vi "Graphe 3D_Qua2ray.vi"(4 "Nbre colonnes":i8=4 min=1, 5 "file path (dialog if empty)":path caption="chemin du fichier (boîte de dialogue si vide)", 7 "Nbre lignes entête":i8=2 min=1, 8 "N° colonne Y":i8=2 min=1, 9 "N° colonne X":i8=1 min=1) -> ()   [LabVIEW 2013]
uses:
  <vilib>/Platform/NI_3dgraph.lvlib
  <vilib>/Analysis/NI_AALBase.lvlib
panel:
  out "Go":bool
  in  "Init Vue":bool
  in  "Plan - Vue":i32(ring)=3 items=["Plan XY", "Plan XZ", "Plan YZ", "Vue 3D"]
  in  "System Link Text 4":bool
  in  "System Link Text 3":bool
  out "Ecart type":dbl caption="Ecart-type" format="%0.2f"
  in  "System Link Text 2":bool
  in  "System Link Text":bool
  out "Min":dbl
  out "Max":dbl
  out "Moyenne":dbl format="%0.2f"
  in  "Inverser échelle Y":bool caption="Y"
  in  "Inverser échelle x":bool caption="X"
  in  "Plot Style":i32(ring)=5 caption="Style de courbe" items=["Ligne"=1, "Point"=2, "Ligne - Point"=3, "Maillage"=4, "Surface"=5, "Surface - Ligne"=6, "Surface Normale"=7, "Contour Ligne"=8, "Surface Contour"=9]
  in  "Transparency (%)":dbl(slide) caption="Transparence (%)" scale=0.0..80.0
  in  "Quit":bool
  in  "Paramètre":u16(ring)
  in  "3D Surface 4":refnum<k7>(container) caption="Surface en 3D"
  in  "3D Surface 3":refnum<k7>(container) caption="Surface en 3D"
  in  "3D Surface 2":refnum<k7>(container) caption="Surface en 3D"
  in  "3D Surface":refnum<k7>(container) caption="Surface en 3D"
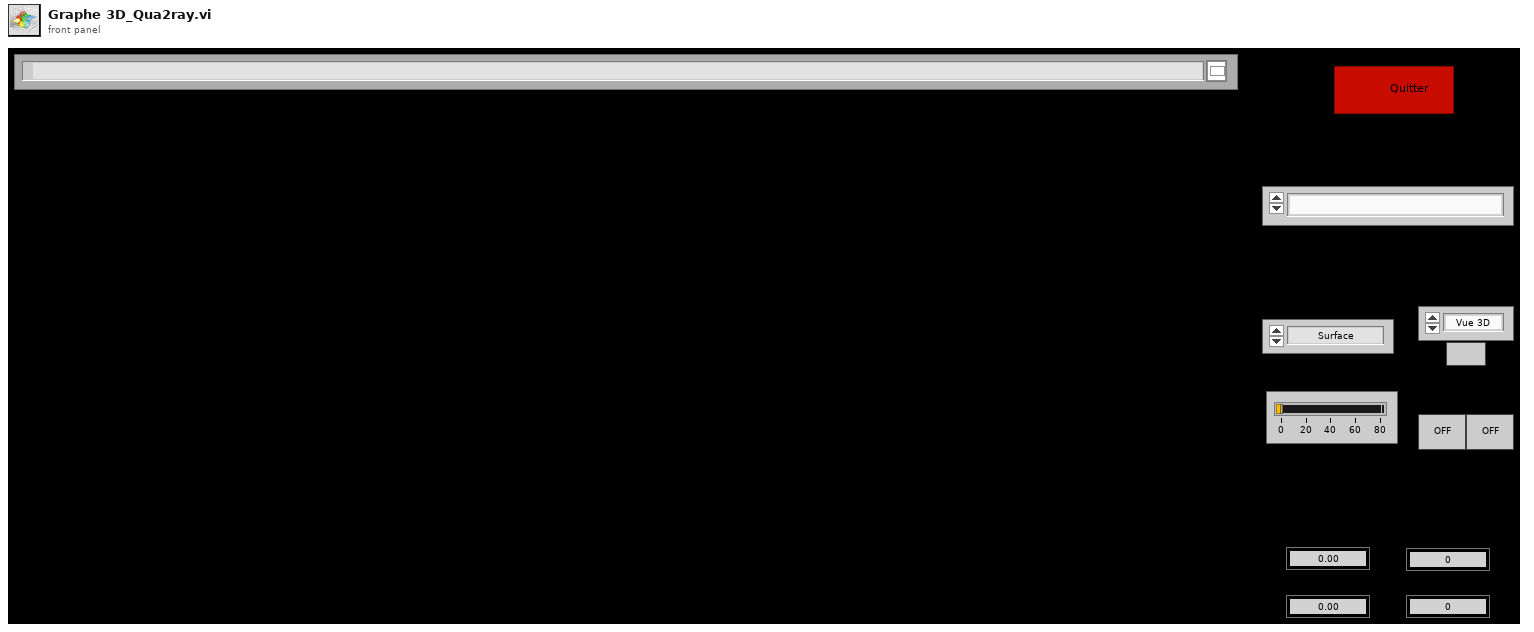
[diagram p1: front panel]
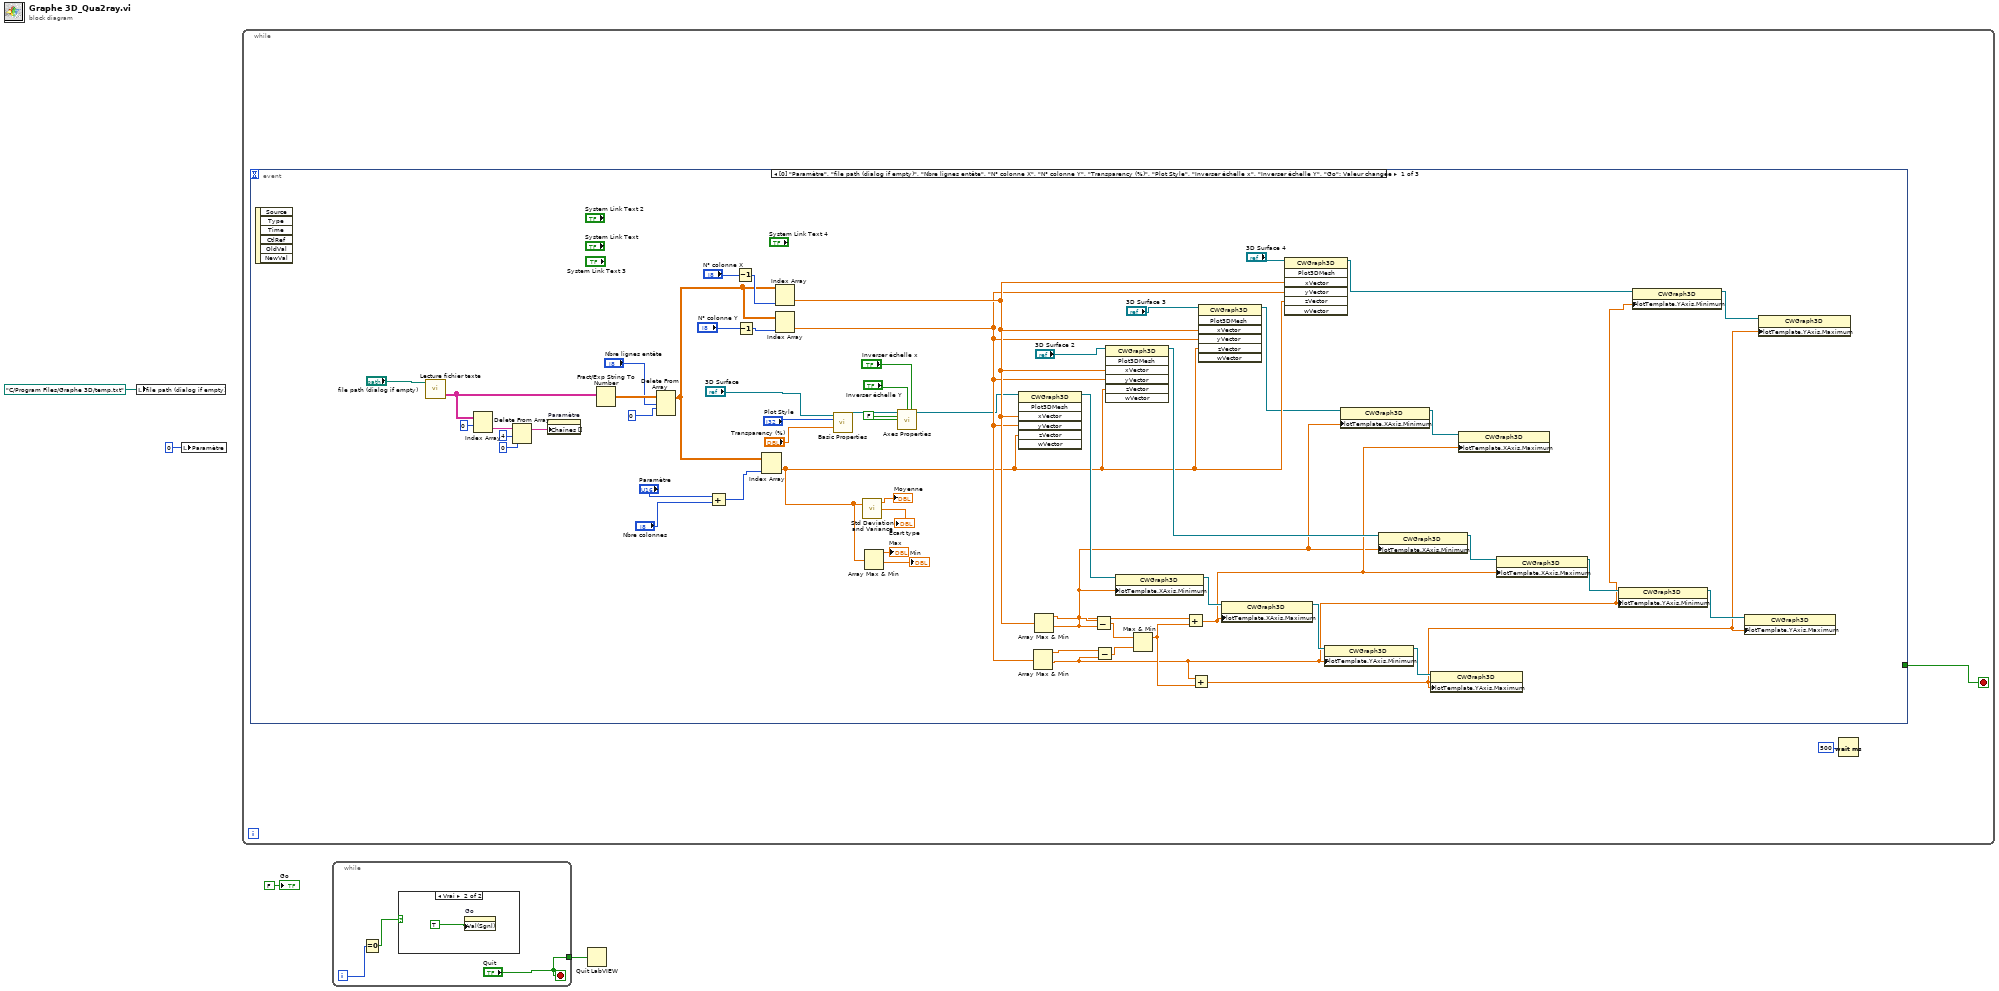
[diagram p0: block diagram]
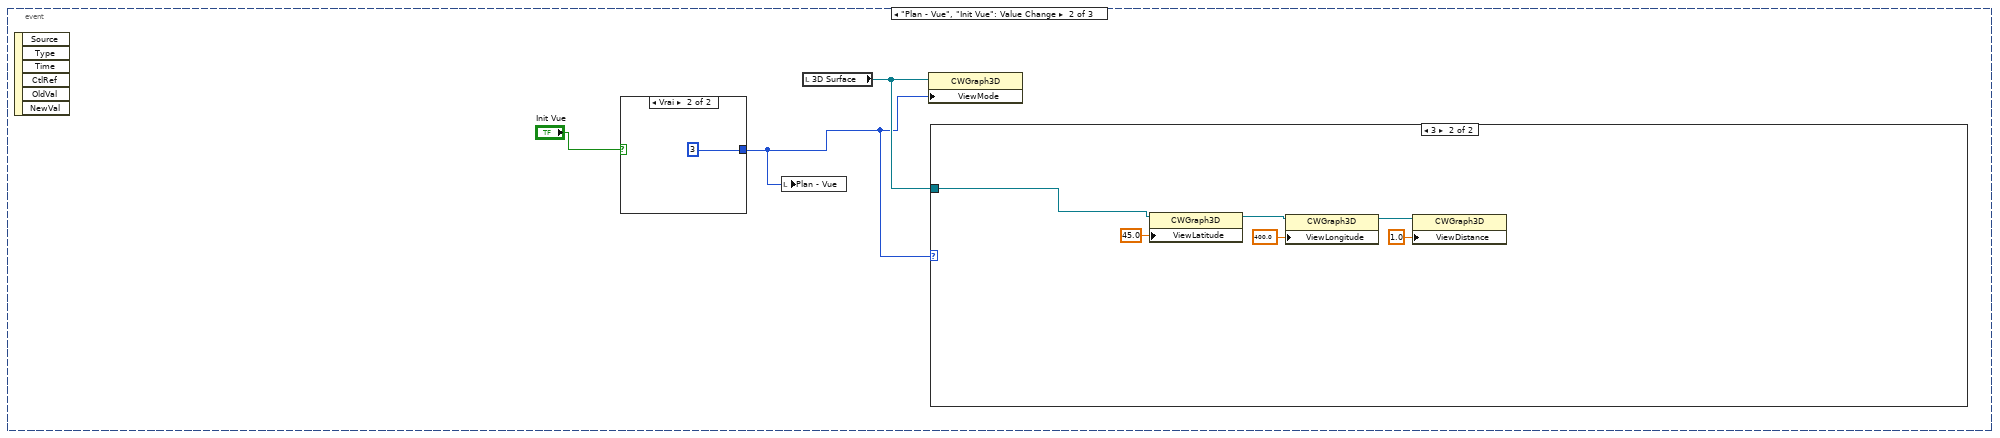
[diagram p3: hidden frame]
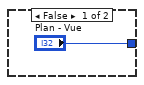
[diagram p4: hidden frame]
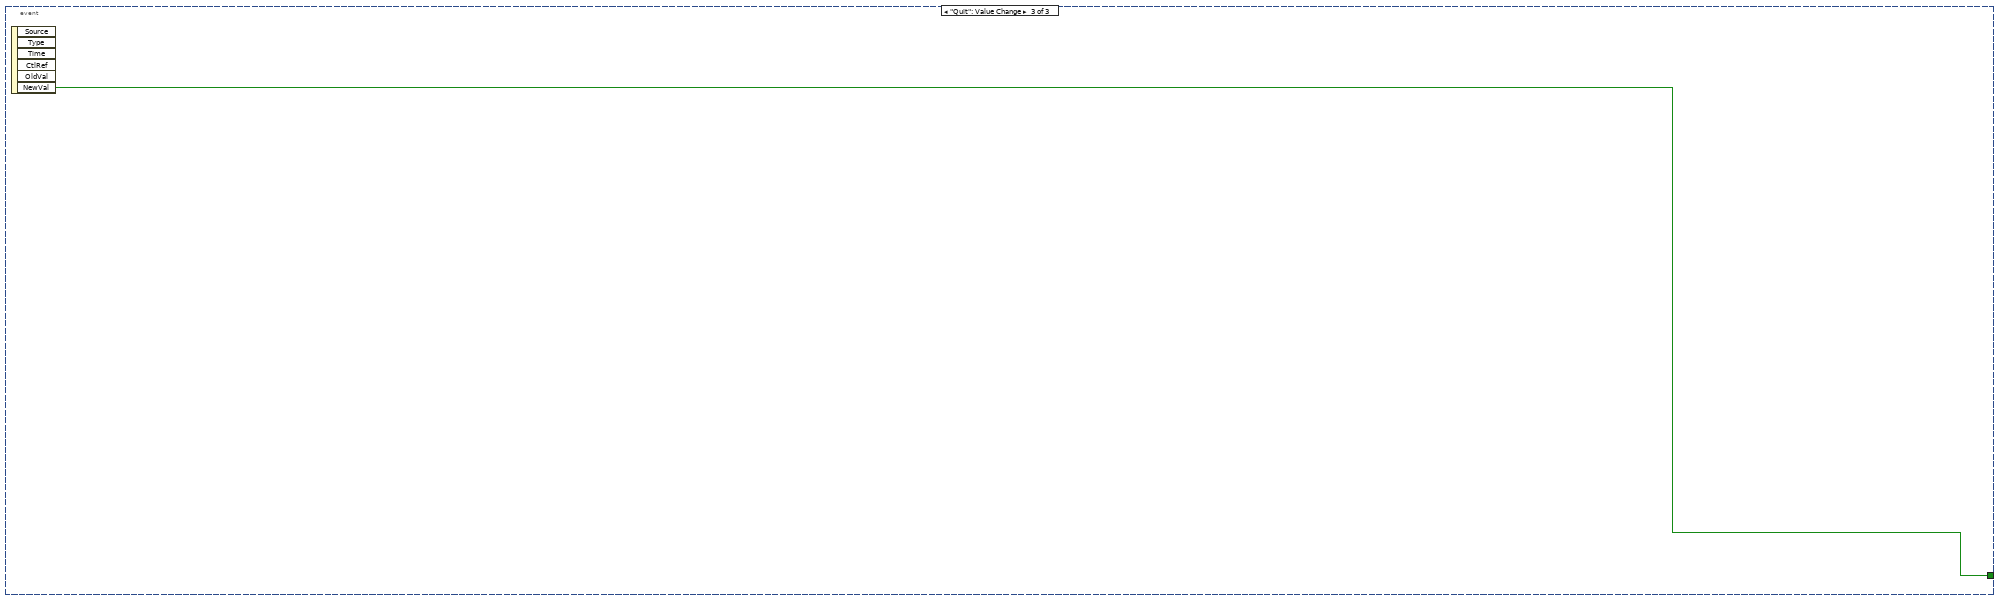
[diagram p6: hidden frame]
diagram:
  n1 = local write "file path (dialog if empty)"(path "C:/Program Files/Graphe 3D/temp.txt" ("file path (dialog if empty)")) -> ()
  n2 = local write "Paramètre"(0) -> ()
  n3 = while {
    stop <- w5 stop-if-true
    n4 = event shown="[0] \"Paramètre\", \"file path (dialog if empty)\", \"Nbre lignes entête\", \"N° colonne X\", \"N° colonne Y\", \"Transparency (%)\", \"Plot Style\", \"Inverser échelle x\", \"Inverser échelle Y\", \"Go\": Valeur changée" {
      selector: _ -> [_ _ _]
      dyn-events: _ -> [_ _ _]
      timeout: _ -> [_ _ _]
      tunnel: [_ _ w75] -> w5
      event "Paramètre", "file path (dialog if empty)", "Nbre lignes entête", "N° colonne X", "N° colonne Y", "Transparency (%)", "Plot Style", "Inverser échelle x", "Inverser échelle Y", "Go": Value Change {
        w40 = FALSE ("auto scale x")
        n5 = event-data() -> ()  [unwired: 1 in, 6 out]
        n6 = call "Lecture fichier texte.vi"("file path (dialog if empty)"="file path (dialog if empty)") -> ("Table"=w11:string[][])  [unwired: 2 in, 1 out]
        n7 = Index Array(array=w11, index (row)=0 ("indice (ligne)")) -> (element=w10:string[])  [unwired: 1 in]
        n8 = Delete From Array(array=w10, length=4 ("longueur"), index=0 ("indice")) -> (array with subset deleted=w9:string[])  [unwired: 1 out]
        n9 = property on="Paramètre" class="MDér (strict)"("Chaînes []"=w9) -> ()  [unwired: 2 in, 2 out]
        n10 = Fract/Exp String To Number(string=w11) -> (number=w62:dbl[][])  [unwired: 3 in, 1 out]
        n11 = Delete From Array(array=w62, length="Nbre lignes entête", index (row)=0 ("indice (ligne)")) -> (array with subset deleted=w46:dbl[][])  [unwired: 1 in, 1 out]
        n12 = Add(x="Paramètre", y="Nbre colonnes") -> (x+y=w14:u16)
        n13 = Decrement(x="N° colonne X") -> (x-1=w57:i8)
        n14 = Decrement(x="N° colonne Y") -> (x-1=w59:i8)
        n15 = Index Array(array=w46, index (col)=w14) -> (element=w27:dbl[])  [unwired: 1 in]
        n16 = Index Array(array=w46, index (col)=w57) -> (element=w45:dbl[])  [unwired: 1 in]
        n17 = Index Array(array=w46, index (col)=w59) -> (element=w44:dbl[])  [unwired: 1 in]
        n18 = call <vilib>:"Basic Properties.vi"("3D graph"="3D Surface", "plot style"="Plot Style", "transparency"="Transparency (%)") -> ("3D graph out"=w56:refnum<k7>)  [unwired: 11 in, 1 out]
        n19 = call <vilib>:"Std Deviation and Variance.vi"("X"=w27) -> ("mean"=→"Moyenne":dbl, "standard deviation"=→"Ecart type":dbl)  [unwired: 1 in, 1 out]
        n20 = Array Max & Min(array=w27) -> (max value=→"Max":dbl, min value=→"Min":dbl)  [unwired: 2 out]
        n21 = call <vilib>:"Axes Properties.vi"("3D graph"=w56, "invert y"="Inverser échelle Y", "invert x"="Inverser échelle x", "auto scale x"=w40, "auto scale y"=w40) -> ("3D graph out"=w34:refnum<k7>)  [unwired: 9 in, 1 out]
        n22 = invoke class="CWGraph3D" method="Plot3DMesh"(reference=w34, "xVector"=w45, "yVector"=w44, "zVector"=w27) -> (reference out=w33:refnum<k7>)  [unwired: 3 in, 6 out]
        n23 = Array Max & Min(array=w44) -> (max value=w37:dbl, min value=w19:dbl)  [unwired: 2 out]
        n24 = Array Max & Min(array=w45) -> (max value=w39:dbl, min value=w17:dbl)  [unwired: 2 out]
        n25 = Subtract(x=w39, y=w17) -> (x-y=w38:dbl)
        n26 = Subtract(x=w37, y=w19) -> (x-y=w36:dbl)
        n27 = invoke class="CWGraph3D" method="Plot3DMesh"(reference="3D Surface 2", "xVector"=w45, "yVector"=w44, "zVector"=w27) -> (reference out=w28:refnum<k7>)  [unwired: 3 in, 6 out]
        n28 = property class="CWGraph3D"(reference=w33, "PlotTemplate.XAxis.Minimum"=w17) -> (reference out=w43:refnum<k7>)  [unwired: 1 in, 1 out]
        n29 = Max & Min(x=w38, y=w36) -> (max(x,y)=w35:dbl)  [unwired: 1 out]
        n30 = Add(x=w17, y=w35) -> (x+y=w18:dbl)
        n31 = Add(x=w19, y=w35) -> (x+y=w20:dbl)
        n32 = invoke class="CWGraph3D" method="Plot3DMesh"(reference="3D Surface 3", "xVector"=w45, "yVector"=w44, "zVector"=w27) -> (reference out=w22:refnum<k7>)  [unwired: 3 in, 6 out]
        n33 = property class="CWGraph3D"(reference=w43, "PlotTemplate.XAxis.Maximum"=w18) -> (reference out=w41:refnum<k7>)  [unwired: 1 in, 1 out]
        n34 = invoke class="CWGraph3D" method="Plot3DMesh"(reference="3D Surface 4", "xVector"=w45, "yVector"=w44, "zVector"=w27) -> (reference out=w21:refnum<k7>)  [unwired: 3 in, 6 out]
        n35 = property class="CWGraph3D"(reference=w41, "PlotTemplate.YAxis.Minimum"=w19) -> (reference out=w42:refnum<k7>)  [unwired: 1 in, 1 out]
        n36 = property class="CWGraph3D"(reference=w22, "PlotTemplate.XAxis.Minimum"=w17) -> (reference out=w24:refnum<k7>)  [unwired: 1 in, 1 out]
        n37 = property class="CWGraph3D"(reference=w28, "PlotTemplate.XAxis.Minimum"=w17) -> (reference out=w31:refnum<k7>)  [unwired: 1 in, 1 out]
        n38 = property class="CWGraph3D"(reference=w42, "PlotTemplate.YAxis.Maximum"=w20) -> ()  [unwired: 1 in, 2 out]
        n39 = property class="CWGraph3D"(reference=w24, "PlotTemplate.XAxis.Maximum"=w18) -> ()  [unwired: 1 in, 2 out]
        n40 = property class="CWGraph3D"(reference=w31, "PlotTemplate.XAxis.Maximum"=w18) -> (reference out=w30:refnum<k7>)  [unwired: 1 in, 1 out]
        n41 = property class="CWGraph3D"(reference=w30, "PlotTemplate.YAxis.Minimum"=w19) -> (reference out=w29:refnum<k7>)  [unwired: 1 in, 1 out]
        n42 = property class="CWGraph3D"(reference=w21, "PlotTemplate.YAxis.Minimum"=w19) -> (reference out=w23:refnum<k7>)  [unwired: 1 in, 1 out]
        n43 = property class="CWGraph3D"(reference=w29, "PlotTemplate.YAxis.Maximum"=w20) -> ()  [unwired: 1 in, 2 out]
        n44 = property class="CWGraph3D"(reference=w23, "PlotTemplate.YAxis.Maximum"=w20) -> ()  [unwired: 1 in, 2 out]
      }
      event "Plan - Vue", "Init Vue": Value Change {
        n45 = event-data() -> ()  [unwired: 1 in, 6 out]
        n46 = case shown="Vrai" "Init Vue" {
          tunnel: ["Plan - Vue" 3 ("Plan - Vue")] -> w64
          frame False {
          }
          frame True {
          }
        }
        n47 = local write "Plan - Vue"(w64) -> ()
        n48 = local read "3D Surface"() -> (w66:refnum<k7>)
        n49 = property class="CWGraph3D"(reference=w66, "ViewMode"=w64) -> ()  [unwired: 1 in, 2 out]
        n50 = case shown="3" w64 {
          tunnel: w66 -> [_ w69]
          frame 0, Default {
          }
          frame 3 {
            n51 = property class="CWGraph3D"(reference=w69, "ViewLatitude"=45.0) -> (reference out=w72:refnum<k7>)  [unwired: 1 in, 1 out]
            n52 = property class="CWGraph3D"(reference=w72, "ViewLongitude"=400.0) -> (reference out=w74:refnum<k7>)  [unwired: 1 in, 1 out]
            n53 = property class="CWGraph3D"(reference=w74, "ViewDistance"=1.0) -> ()  [unwired: 1 in, 2 out]
          }
        }
      }
      event "Quit": Value Change {
        n54 = event-data() -> ("NewVal"=w75:bool)  [unwired: 1 in, 5 out]
      }
    }
    n55 = Wait (ms)(milliseconds to wait=u32 500 ("attente (ms)")) -> ()  [unwired: 1 out]
  }
  n56 = while {
    tunnel: ["Quit"] -> w1
    i -> [w77]
    stop <- "Quit" stop-if-true
    n57 = Equal To 0?(x=w77) -> (x = 0?=w78:bool)
    n58 = case shown="Vrai" w78 {
      frame False {
      }
      frame True {
        n59 = property on="Go" class="Bool"("Val(Sgnl)"=TRUE) -> ()  [unwired: 2 in, 2 out]
      }
    }
  }
  n60 = Quit LabVIEW(quit? (T)=w1) -> ()
  "Go" <- FALSE ("Go")
